vi "Pack PII Error_Graph_v00.vi"(5 "PII+Error pump A":T4, 7 "PII+Error pump B":T4, 8 "PII+Error HD B":T8, 9 "PII+Error HD A":T8, 10 "PII+Error Graph BS":T4, 11 "PII+Error EPR BS":T4) -> (0 "Theta":T2, 1 "Thresholds":cluster{"Lock":T7, "Re-Scan":T7}, 3 "Error packed":T3={"Pre-Offset"={"Pre-Offset 1"=2, "Pre-Offset 2"=0, "Pre-Offset 3"=0, "Pre-Offset 4"=0, "Pre-Offset 5"=2, "Pre-Offset 6"=0, "Pre-Offset 7"=0, "Pre-Offset 8"=0}, "Post-Offset "={"Offset 1"=0, "Offset 2"=0, "Offset 3"=0, "Offset 4"=0, "Offset 5"=0, "Offset 6"=0, "Offset 7"=0, "Offset 8"=0}, "Gains"={"Gain 1"=0, "Gain 2"=0, "Gain 3"=0, "Gain 4"=0, "Gain 5"=0, "Gain 6"=0, "Gain 7"=0, "Gain 8"=0}, "Bit Shifts"={"Bit Shift 1"=0, "Bit Shift 2"=300, "Bit Shift 3"=0, "Bit Shift 4"=0, "Bit Shift 5"=0, "Bit Shift 6"=0, "Bit Shift 7"=0, "Bit Shift 8"=0}})   [LabVIEW 2010]
doc: "Packages individual values related to error signal scaling from the user interface into data structures compatible with FPGA_Cavities.VI\n(very messy, could use a tidy)."
uses:
  Strict Type Defs/Graph Errors I16.ctl
  Strict Type Defs/Error Scale Graph.ctl
  Strict Type Defs/PII and Error Graph.ctl
  Strict Type Defs/Errors Converted Graph.ctl
  Strict Type Defs/PII individual.ctl
  Strict Type Defs/PII and Error Graph HD.ctl
  Strict Type Defs/Errors Converted Graph HD.ctl
  Strict Type Defs/Lock Thresh Graph.ctl
  Strict Type Defs/Theta graph.ctl
panel:
  in  "Bit Shifts":T1
  in  "Theta typedef":T2
  in  "Error scale graph type":T3={"Pre-Offset"={"Pre-Offset 1"=2, "Pre-Offset 2"=0, "Pre-Offset 3"=0, "Pre-Offset 4"=0, "Pre-Offset 5"=2, "Pre-Offset 6"=0, "Pre-Offset 7"=0, "Pre-Offset 8"=0}, "Post-Offset "={"Offset 1"=0, "Offset 2"=300, "Offset 3"=0, "Offset 4"=0, "Offset 5"=0, "Offset 6"=0, "Offset 7"=0, "Offset 8"=0}, "Gains"={"Gain 1"=0, "Gain 2"=300, "Gain 3"=0, "Gain 4"=0, "Gain 5"=0, "Gain 6"=0, "Gain 7"=0, "Gain 8"=0}, "Bit Shifts"={"Bit Shift 1"=0, "Bit Shift 2"=300, "Bit Shift 3"=0, "Bit Shift 4"=0, "Bit Shift 5"=0, "Bit Shift 6"=0, "Bit Shift 7"=0, "Bit Shift 8"=0}}
  in  "Thresholds type def":cluster{"Lock":T7, "Re-Scan":T7}
  in  "Re-Scan Thresh":T7
  in  "Lock Thresh":T7
  in  "Pre Offset":T1
  in  "Offset":T1
  in  "Gains":T1
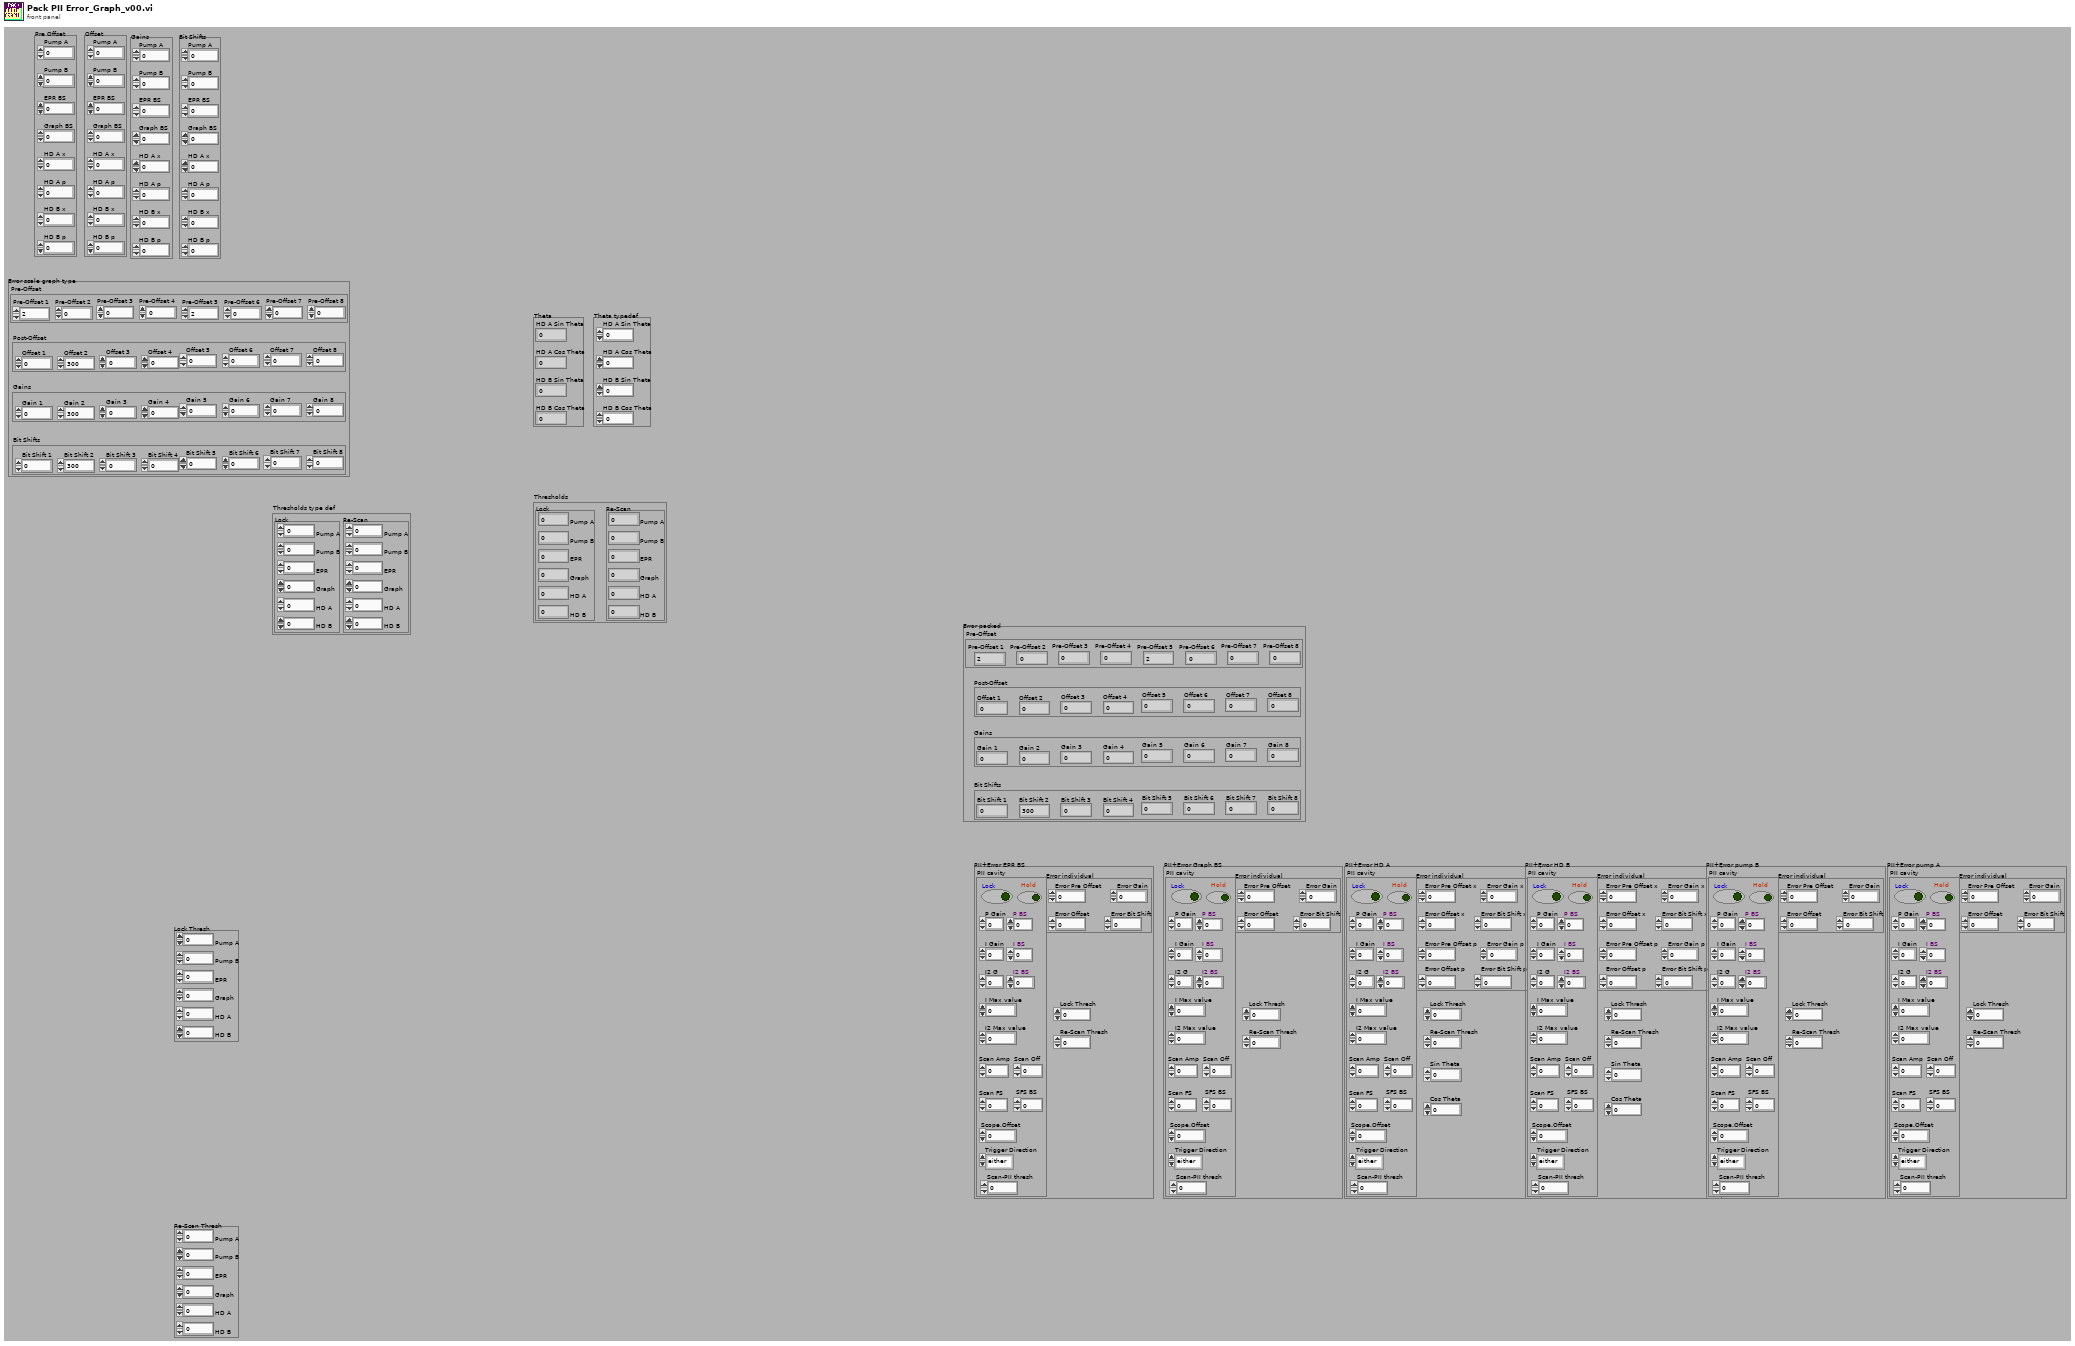
[diagram p1: front panel]
types:
  T1 = typedef "Graph Errors I16.ctl" = cluster{"Pump A":i16, "Pump B":i16, "EPR BS":i16, "Graph BS":i16, "HD A x":i16, "HD A p":i16, "HD B x":i16, "HD B p":i16}
  T2 = typedef "Theta graph.ctl" = cluster{"HD A Sin Theta":i32, "HD A Cos Theta":i32, "HD B Sin Theta":i32, "HD B Cos Theta":i32}
  T3 = typedef "Error Scale Graph.ctl" = cluster{"Pre-Offset":cluster{"Pre-Offset 1":i16, "Pre-Offset 2":i16, "Pre-Offset 3":i16, "Pre-Offset 4":i16, "Pre-Offset 5":i16, "Pre-Offset 6":i16, "Pre-Offset 7":i16, "Pre-Offset 8":i16}, "Post-Offset ":cluster{"Offset 1":i16, "Offset 2":i16, "Offset 3":i16, "Offset 4":i16, "Offset 5":i16, "Offset 6":i16, "Offset 7":i16, "Offset 8":i16}, "Gains":cluster{"Gain 1":i16, "Gain 2":i16, "Gain 3":i16, "Gain 4":i16, "Gain 5":i16, "Gain 6":i16, "Gain 7":i16, "Gain 8":i16}, "Bit Shifts":cluster{"Bit Shift 1":i16, "Bit Shift 2":i16, "Bit Shift 3":i16, "Bit Shift 4":i16, "Bit Shift 5":i16, "Bit Shift 6":i16, "Bit Shift 7":i16, "Bit Shift 8":i16}}
  T4 = typedef "PII and Error Graph.ctl" = cluster{"Error individual":T5, "PII cavity":T6, "Lock Thresh":i16, "Re-Scan Thresh":i16}
  T5 = typedef "Errors Converted Graph.ctl" = cluster{"Error Pre Offset":i16, "Error Offset":i16, "Error Gain":i16, "Error Bit Shift":i16}
  T6 = typedef "PII individual.ctl" = cluster{"Lock":bool, "Hold":bool, "P Gain":i32, "P BS":i16, "I Gain":i32, "I BS":i16, "I2 G":i32, "I2 BS":i16, "Scan Amp":i16, "Scan Off":i16, "Scan FS":u16, "SFS BS":i16, "I Max value":i32, "I2 Max value":i32, "Scope.Offset":i16, "Trigger Direction":enum8{"either", "minus-plus", "plus-minus"}, "Scan-PII thresh":i16}
  T7 = typedef "Lock Thresh Graph.ctl" = cluster{"Pump A":i16, "Pump B":i16, "EPR":i16, "Graph":i16, "HD A":i16, "HD B":i16}
  T8 = typedef "PII and Error Graph HD.ctl" = cluster{"Error individual":T9, "PII cavity":T6, "Lock Thresh":i16, "Re-Scan Thresh":i16, "Sin Theta":i32, "Cos Theta":i32}
  T9 = typedef "Errors Converted Graph HD.ctl" = cluster{"Error Pre Offset x":i16, "Error Offset x":i16, "Error Gain x":i16, "Error Bit Shift x":i16, "Error Pre Offset p":i16, "Error Offset p":i16, "Error Gain p":i16, "Error Bit Shift p":i16}
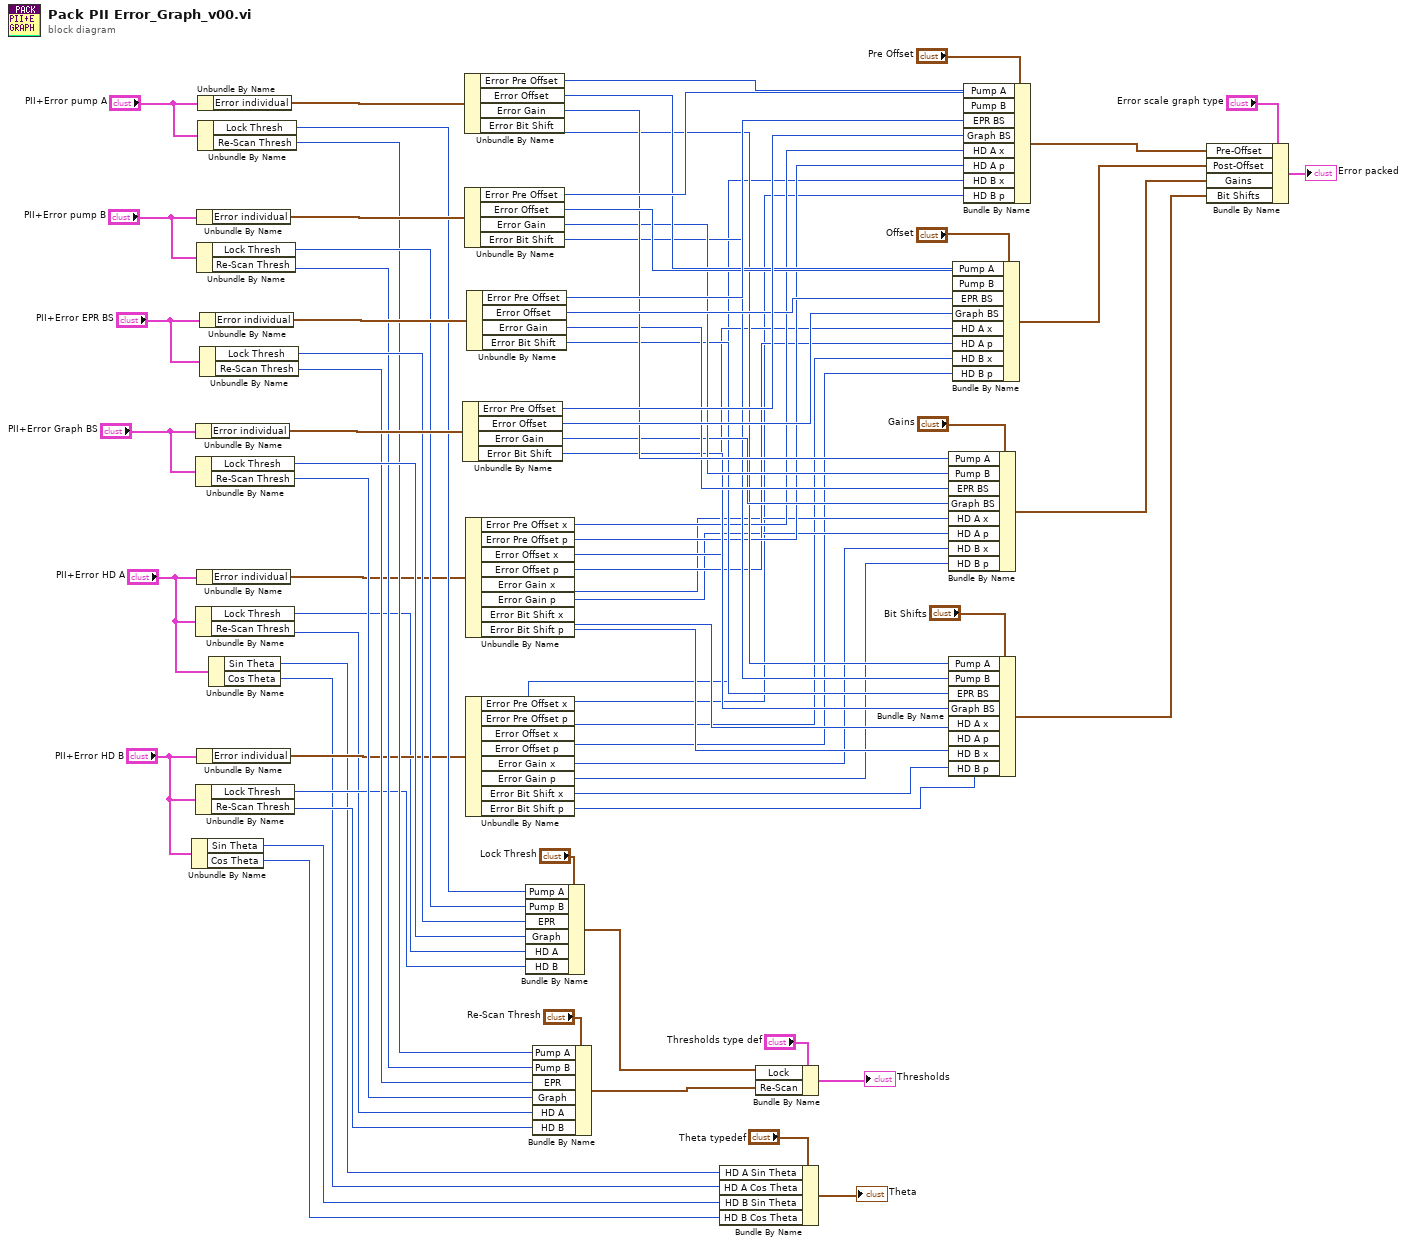
[diagram p0: block diagram]
diagram:
  n1 = Unbundle By Name("PII+Error HD B") -> ("Sin Theta"=w2:i32, "Cos Theta"=w1:i32)
  n2 = Unbundle By Name("PII+Error Graph BS") -> ("Error individual"=w75:T5)
  n3 = Unbundle By Name("PII+Error Graph BS") -> ("Lock Thresh"=w51:i16, "Re-Scan Thresh"=w46:i16)
  n4 = Unbundle By Name("PII+Error HD A") -> ("Lock Thresh"=w10:i16, "Re-Scan Thresh"=w8:i16)
  n5 = Unbundle By Name("PII+Error HD B") -> ("Lock Thresh"=w9:i16, "Re-Scan Thresh"=w7:i16)
  n6 = Unbundle By Name("PII+Error pump B") -> ("Error individual"=w76:T5)
  n7 = Unbundle By Name("PII+Error pump B") -> ("Lock Thresh"=w53:i16, "Re-Scan Thresh"=w48:i16)
  n8 = Unbundle By Name("PII+Error HD A") -> ("Error individual"=w28:T9)
  n9 = Unbundle By Name("PII+Error HD B") -> ("Error individual"=w19:T9)
  n10 = Unbundle By Name("PII+Error pump A") -> ("Error individual"=w77:T5)
  n11 = Unbundle By Name("PII+Error pump A") -> ("Lock Thresh"=w54:i16, "Re-Scan Thresh"=w49:i16)
  n12 = Unbundle By Name("PII+Error EPR BS") -> ("Error individual"=w74:T5)
  n13 = Unbundle By Name("PII+Error EPR BS") -> ("Lock Thresh"=w52:i16, "Re-Scan Thresh"=w47:i16)
  n14 = Unbundle By Name("PII+Error HD A") -> ("Sin Theta"=w5:i32, "Cos Theta"=w4:i32)
  n15 = Unbundle By Name(w75) -> ("Error Pre Offset"=w70:i16, "Error Offset"=w66:i16, "Error Gain"=w62:i16, "Error Bit Shift"=w29:i16)
  n16 = Unbundle By Name(w77) -> ("Error Pre Offset"=w73:i16, "Error Offset"=w69:i16, "Error Gain"=w65:i16, "Error Bit Shift"=w32:i16)
  n17 = Unbundle By Name(w76) -> ("Error Pre Offset"=w72:i16, "Error Offset"=w68:i16, "Error Gain"=w64:i16, "Error Bit Shift"=w31:i16)
  n18 = Unbundle By Name(w28) -> ("Error Pre Offset x"=w27:i16, "Error Pre Offset p"=w26:i16, "Error Offset x"=w25:i16, "Error Offset p"=w24:i16, "Error Gain x"=w23:i16, "Error Gain p"=w22:i16, "Error Bit Shift x"=w21:i16, "Error Bit Shift p"=w20:i16)
  n19 = Unbundle By Name(w19) -> ("Error Pre Offset x"=w11:i16, "Error Pre Offset p"=w12:i16, "Error Offset x"=w13:i16, "Error Offset p"=w14:i16, "Error Gain x"=w15:i16, "Error Gain p"=w16:i16, "Error Bit Shift x"=w17:i16, "Error Bit Shift p"=w18:i16)
  n20 = Unbundle By Name(w74) -> ("Error Pre Offset"=w71:i16, "Error Offset"=w67:i16, "Error Gain"=w63:i16, "Error Bit Shift"=w30:i16)
  n21 = Bundle By Name(cluster="Lock Thresh", "Pump A"=w54, "Pump B"=w53, "EPR"=w52, "Graph"=w51, "HD A"=w10, "HD B"=w9) -> (w44:T7)
  n22 = Bundle By Name(cluster="Re-Scan Thresh", "Pump A"=w49, "Pump B"=w48, "EPR"=w47, "Graph"=w46, "HD A"=w8, "HD B"=w7) -> (w43:T7)
  n23 = Bundle By Name(cluster="Theta typedef", "HD A Sin Theta"=w5, "HD A Cos Theta"=w4, "HD B Sin Theta"=w2, "HD B Cos Theta"=w1) -> (→"Theta":T2)
  n24 = Bundle By Name(cluster="Thresholds type def", "Lock"=w44, "Re-Scan"=w43) -> (→"Thresholds":cluster{"Lock":T7, "Re-Scan":T7})
  n25 = Bundle By Name(cluster="Gains", "Pump A"=w65, "Pump B"=w64, "EPR BS"=w63, "Graph BS"=w62, "HD A x"=w23, "HD A p"=w22, "HD B x"=w15, "HD B p"=w16) -> (w58:T1)
  n26 = Bundle By Name(cluster="Bit Shifts", "Pump A"=w32, "Pump B"=w31, "EPR BS"=w30, "Graph BS"=w29, "HD A x"=w21, "HD A p"=w20, "HD B x"=w17, "HD B p"=w18) -> (w37:T1)
  n27 = Bundle By Name(cluster="Offset", "Pump A"=w69, "Pump B"=w68, "EPR BS"=w67, "Graph BS"=w66, "HD A x"=w25, "HD A p"=w24, "HD B x"=w13, "HD B p"=w14) -> (w56:T1)
  n28 = Bundle By Name(cluster="Pre Offset", "Pump A"=w73, "Pump B"=w72, "EPR BS"=w71, "Graph BS"=w70, "HD A x"=w27, "HD A p"=w26, "HD B x"=w11, "HD B p"=w12) -> (w61:T1)
  n29 = Bundle By Name(cluster="Error scale graph type", "Pre-Offset"=w61, "Post-Offset"=w56, "Gains"=w58, "Bit Shifts"=w37) -> (→"Error packed":T3)
